vi "testOccurrenceDll.vi"() -> ()   [LabVIEW 2011]
panel:
  out "Occurrence":i32
  in  "布尔":bool
  out "数值 2":i32
  out "数值":i32
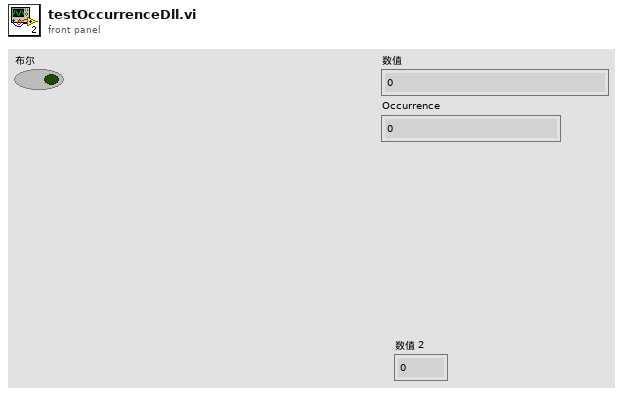
[diagram p1: front panel]
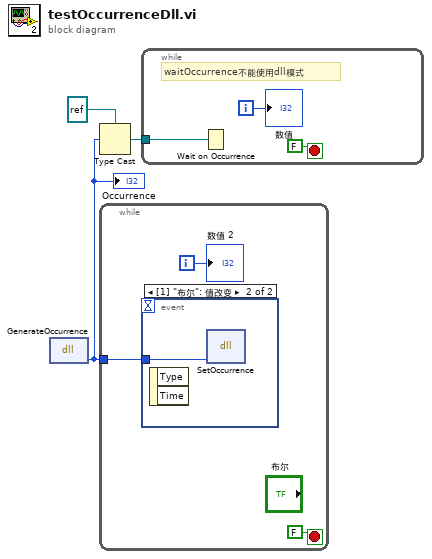
[diagram p0: block diagram]
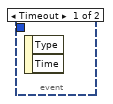
[diagram p2: hidden frame]
diagram:
  n1 = dll-call lib="PTH1Labs GworkLuaDllToLabviewbuilds\ttestC_dll\t我的DLLOccurrence.dll" fn="GenerateOccurrence"() -> ("返回类型"=w1:i32)  [unwired: 3 in, 2 out]
  "Occurrence" <- w1
  n2 = Type Cast(type=refnum<k4> refnum ("事件发生"), x=w1) -> (*(type *) &x=w2:refnum<k4>)
  n3 = while {
    tunnel: w1 -> [w4]
    i -> [w5]
    stop <- FALSE stop-if-true
    n4 = event shown="[1] \"布尔\": 值改变" {
      selector: _ -> [_ _]
      dyn-events: _ -> [_ _]
      timeout: _ -> [_ _]
      tunnel: w4 -> [_ w7]
      event Timeout {
        n5 = event-data() -> ()  [unwired: 1 in, 2 out]
      }
      event "布尔": Value Change {
        n6 = event-data() -> ()  [unwired: 1 in, 2 out]
        n7 = dll-call lib="PTH1Labs GworkLuaDllToLabviewbuilds\ttestC_dll\t我的DLLOccurrence.dll" fn="SetOccurrence"("occurence"=w7) -> ()  [unwired: 5 in, 2 out]
      }
    }
    "数值 2" <- w5
  }
  n8 = while {
    tunnel: w2 -> [w8]
    i -> [w9]
    stop <- FALSE stop-if-true
    # "waitOccurrence不能使用dll模式"
    n9 = Wait on Occurrence(2:w8) -> ()  [unwired: 2 in, 1 out]
    "数值" <- w9
  }
